vi "toml_load_comment.vi"(8 "error in (no error)":errorcluster, 11 "toml":string) -> (0 "error out":errorcluster, 2 "remaining string":string, 3 "inline comment":string)   [LabVIEW 2017]
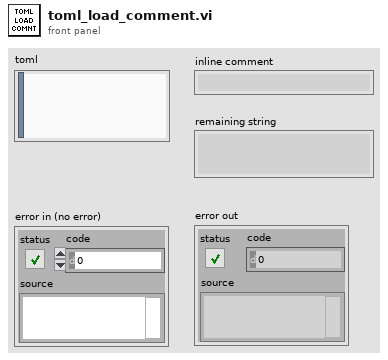
[diagram p1: front panel]
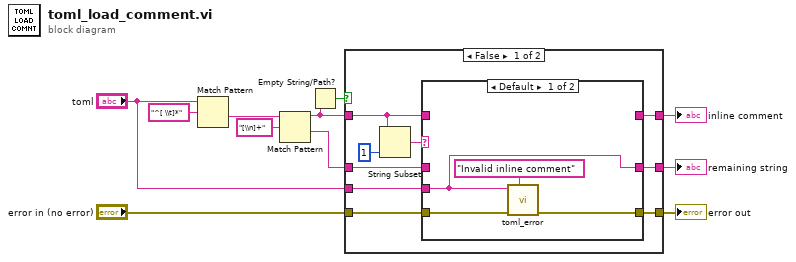
[diagram p0: block diagram]
diagram:
  n1 = Match Pattern(string="toml", regular expression="^[ \\t]*") -> (after substring=w5:string)  [unwired: 1 in, 3 out]
  n2 = Match Pattern(string=w5, regular expression="[\\n]+") -> (before substring=w8:string, after substring=w1:string)  [unwired: 1 in, 2 out]
  n3 = Empty String/Path?(string/path=w8) -> (empty?=w7:bool)
  n4 = case shown="False" w7 {
    tunnel: w8 -> [w14 _]
    tunnel: "error in (no error)" -> [w20 w28]
    tunnel: [w19 w28] -> w9
    tunnel: "toml" -> [w16 _]
    tunnel: [w15 _] -> w3
    tunnel: [w13 w29] -> w2
    tunnel: w1 -> [w12 w29]
    frame False {
      n5 = String Subset(string=w14, length (rest)=1 ("length (rest)")) -> (substring=w18:string)  [unwired: 1 in]
      n6 = case shown="Default" w18 {
        tunnel: w20 -> [w24 w27]
        tunnel: [w23 w27] -> w19
        tunnel: w16 -> [w21 _]
        tunnel: [_ w26] -> w15
        tunnel: w14 -> [_ w26]
        tunnel: [w21 w25] -> w13
        tunnel: w12 -> [_ w25]
        frame Default {
          n7 = call "toml_error.vi"("message"="Invalid inline comment", "error in (no error)"=w24, "toml"=w21) -> ("error out"=w23:errorcluster)  [unwired: 8 in]
        }
        frame "#" {
        }
      }
    }
    frame True {
    }
  }
  "remaining string" <- w2
  "inline comment" <- w3
  "error out" <- w9
